vi "Set RTDriver VIs File Paths.vi"(8 "error in (no error)":errorcluster, 11 "Item Ref in":T1 format="%.0x") -> (0 "error out":errorcluster, 3 "Item Ref out":T1 format="%.0x")   [LabVIEW 2019, in "TemplatePPL System Explorer.lvlib"]
uses:
  TemplatePPL System Explorer.lvlib
  <vilib>/NI VeriStand/Custom Device API/Custom Device Item Ref.ctl
  <vilib>/NI VeriStand/Custom Device API/Custom Device API.lvlib
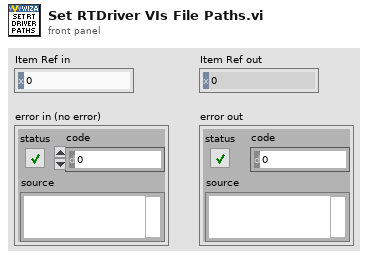
[diagram p1: front panel]
types:
  T1 = typedef "Custom Device API.lvlib/Custom Device Item Ref.ctl" = u64
  T2 = typedef "Advanced System Definition.lvlib/Property.DependentFile.ctl" = cluster{"Original Path":path, "Version":string, "RTDestination":path, "ForceDownload":bool, "SupportedTarget":string, "MD5":string}
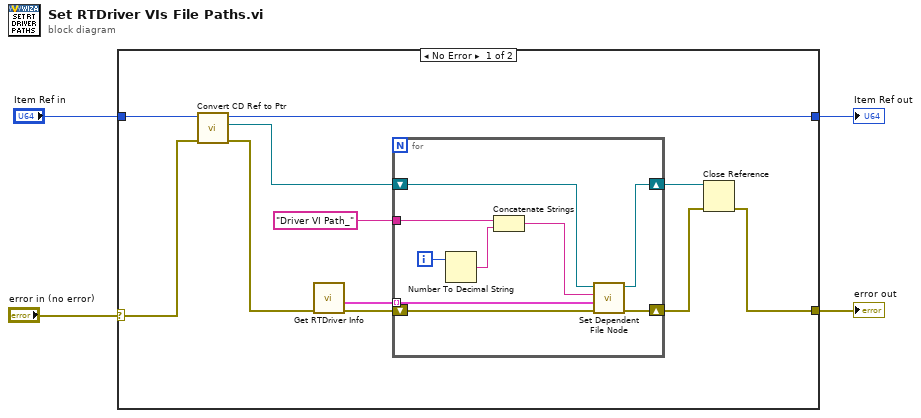
[diagram p0: block diagram]
diagram:
  n1 = case shown="No Error" "error in (no error)" {
    selector: "error in (no error)" -> [w10 w25]
    tunnel: [w14 w25] -> w4
    tunnel: [w8 w26] -> w3
    tunnel: "Item Ref in" -> [w11 w26]
    frame No Error {
      n2 = call "Convert CD Ref to Ptr.vi"("error in (no error)"=w10, "Item Ref in"=w11) -> ("error out"=w7:errorcluster, ".NET Refnum out"=w9:refnum<k24>, "Item Ref out"=w8:T1)  [unwired: 7 in]
      n3 = call "Get RTDriver Info.vi"("error in (no error)"=w7) -> ("error out"=w6:errorcluster, "RT Driver Info"=w5:T2[])  [unwired: 9 in]
      n4 = for {
        shift-right: [w20] -> w13
        shift-left: w6 -> [w21]
        tunnel: w5 -> [w19] mode=indexing
        tunnel: "Driver VI Path_" ("Property name") -> [w24]
        shift-right: [w16] -> w15
        shift-left: w9 -> [w17]
        i -> [w22]
        n5 = Number To Decimal String(number=w22) -> (decimal integer string=w23:string)  [unwired: 1 in]
        n6 = Concatenate Strings(w24, w23) -> (w18:string)
        n7 = call "Set Dependent File Node.vi"("error in (no error)"=w21, "Dependent File info"=w19, "Property name"=w18, ".NET Refnum in"=w17) -> ("error out"=w20:errorcluster, ".NET Refnum out"=w16:refnum<k24>)  [unwired: 5 in, 1 out]
      }
      n8 = Close Reference(reference=w15, error in (no error)=w13) -> (error out=w14:errorcluster)
    }
    frame Error {
    }
  }
  "error out" <- w4
  "Item Ref out" <- w3
